vi "get Pdc Config Ver3.vi"(10 "pseudoPdcId":i32, 11 "pdcCfg":T1) -> (2 "function return":i32, 3 "pdcCfg out":T1)   [LabVIEW 2018, in "S3DK.lvlib" / "C37118-DLL.lvlib" / "StrongridDLL.lvlib"]
doc: "STRONGRIDIEEEC37118DLL_API int __cdecl getPdcConfig_Ver3(pdcConfiguration* pdcCfg, int32_t pseudoPdcId);"
uses:
  StrongridDLL.lvlib
  <vilib>/builds/S3DK Compiler/My Packed Library/StrongridDLL.dll
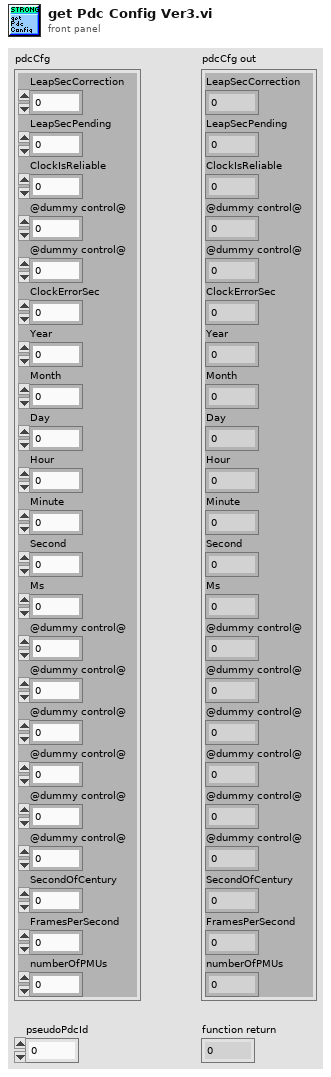
[diagram p1: front panel]
types:
  T1 = cluster{"LeapSecCorrection":i32, "LeapSecPending":u8, "ClockIsReliable":u8, "@dummy control@":i8, "@dummy control@":i8, "ClockErrorSec":sgl, "Year":i16, "Month":i16, "Day":i16, "Hour":i16, "Minute":i16, "Second":i16, "Ms":i16, "@dummy control@":i8, "@dummy control@":i8, "@dummy control@":i8, "@dummy control@":i8, "@dummy control@":i8, "@dummy control@":i8, "SecondOfCentury":dbl, "FramesPerSecond":sgl, "numberOfPMUs":i32}
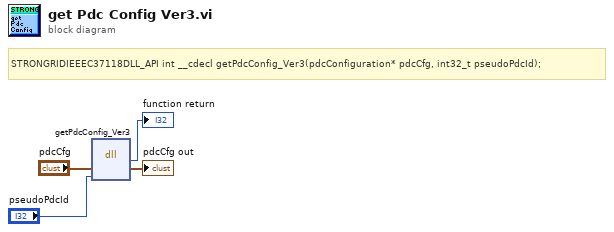
[diagram p0: block diagram]
diagram:
  # "STRONGRIDIEEEC37118DLL_API int __cdecl getPdcConfig_Ver3(pdcConfiguration* pdcCfg, int32_t pseudoPdcId);"
  n1 = dll-call lib="C:/Program Files/National Instruments/LabVIEW 2018/vi.lib/builds/S3DK Compiler/My Packed Library/StrongridDLL.*" fn="getPdcConfig_Ver3"("pdcCfg"="pdcCfg", "pseudoPdcId"="pseudoPdcId") -> (→"function return":i32, "pdcCfg"=→"pdcCfg out":T1)  [unwired: 4 in, 2 out]
